vi "configure.vi"(8 "error in (no error)":errorcluster, 11 "WriteSignalsDAQmxPlugin in":refnum<class "SignalWriterDL090202DAQmx.lvclass">) -> (0 "error out":errorcluster, 3 "WriteSignalsDAQmxPlugin out":refnum<class "SignalWriterDL090202DAQmx.lvclass">)   [LabVIEW 2010, in "SignalWriterDL090202DAQmx.lvclass"]
uses:
  SignalWriterDL090202DAQmx.lvclass
  output_type_enum.ctl
  trigger_edge_enum.ctl
  common/classes/GenericComponent/GenericComponent/GenericComponent.lvclass
panel:
  in  "counter":tag
  out "configuration":string
  in  "edge":T1
  in  "digital trigger line":tag
  in  "output value upper bound":dbl caption="to"
  in  "output value  lower bound":dbl caption="from"
  in  "output type":T2
  in  "maximum sampling rate":dbl[unit]
  in  "lag":dbl[unit]
  in  "timing source":tag
  in  "output physical channel":tag
  in  "cancel button":bool
  in  "save button":bool
  # "Configure DL090202DAQmxWriteSignals"
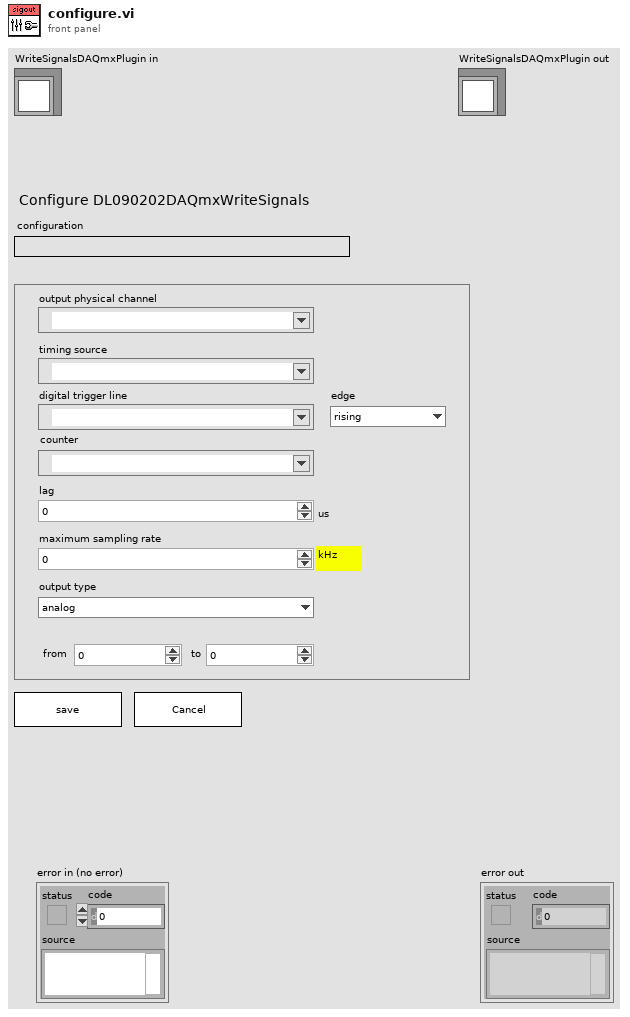
[diagram p1: front panel]
types:
  T1 = typedef "SignalWriterDL090202DAQmx.lvclass/trigger_edge_enum.ctl" = enum16{"rising", "falling"}
  T2 = typedef "SignalWriterDL090202DAQmx.lvclass/output_type_enum.ctl" = enum16{"analog", "digital (U8)", "digital (U16)", "digital (U32)"}
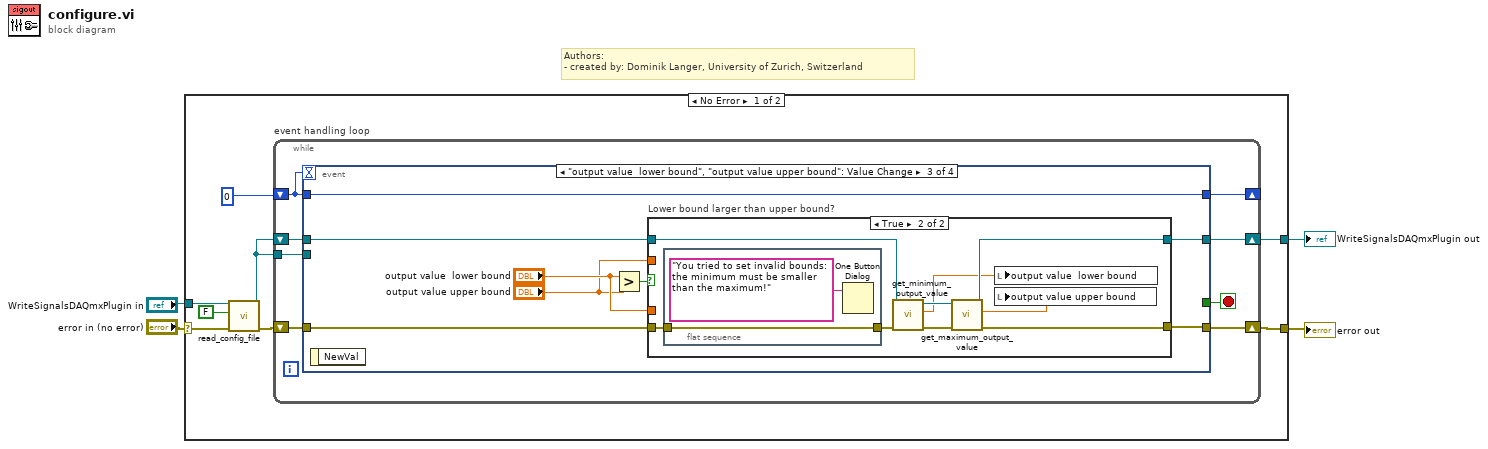
[diagram p0: block diagram]
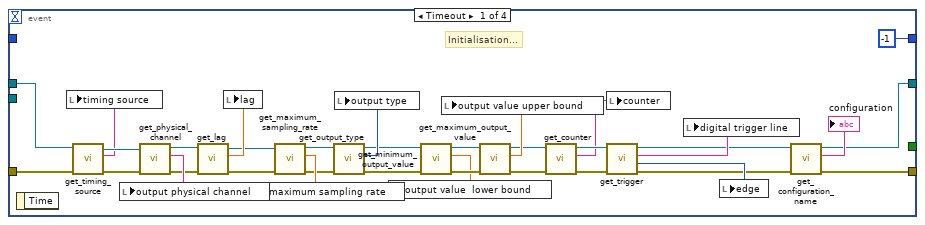
[diagram p2: hidden frame]
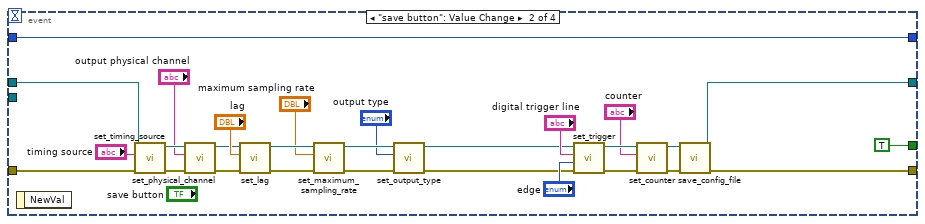
[diagram p3: hidden frame]
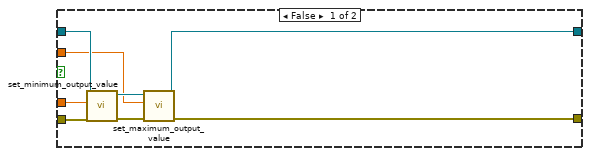
[diagram p4: hidden frame]
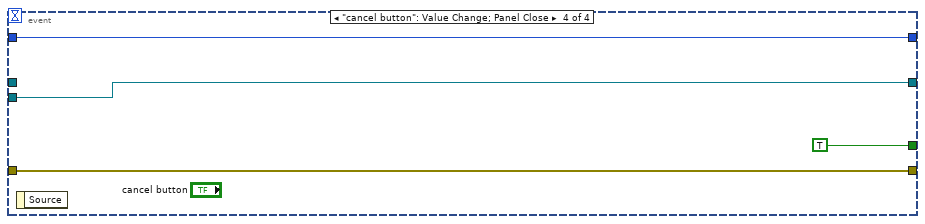
[diagram p5: hidden frame]
diagram:
  # "Authors: \n- created by: Dominik Langer, University of Zurich, Switzerland"
  n1 = case shown="No Error" "error in (no error)" {
    selector: "error in (no error)" -> [w8 w115]
    tunnel: [w12 w115] -> w3
    tunnel: [w10 w114] -> w1
    tunnel: "WriteSignalsDAQmxPlugin in" -> [w9 w114]
    frame No Error {
      n2 = call-dynamic "read_config_file.vi"("error in (no error)"=w8, "force load?"=FALSE, "GenericPlugin in"=w9) -> ("error out"=w7:errorcluster, "GenericPlugin out"=w5:refnum<class "SignalWriterDL090202DAQmx.lvclass">)  [unwired: 7 out]
      n3 = while "event handling loop" {
        shift-right: [w16] -> _
        shift-left: 0 -> [w17]
        shift-right: [w14] -> w10
        shift-left: w5 -> [w15]
        shift-right: [w19] -> w12
        shift-left: w7 -> [w20]
        tunnel: w5 -> [w13]
        stop <- w18 stop-if-true
        n4 = event shown="[2] \"output value  lower bound\", \"output value upper bound\": Value Change" {
          selector: _ -> [_ _ _ _]
          dyn-events: _ -> [_ _ _ _]
          timeout: w17 -> [_ _ _ _]
          tunnel: w20 -> [w34 w79 w89 w112]
          tunnel: [w29 w65 w88 w112] -> w19
          tunnel: [_ TRUE _ TRUE] -> w18
          tunnel: [-1 w82 w90 w111] -> w16
          tunnel: w17 -> [_ w82 w90 w111]
          tunnel: w15 -> [w33 w78 w87 _]
          tunnel: [w26 w64 w86 w110] -> w14
          tunnel: w13 -> [_ _ _ w110]
          event Timeout {
            # "Initialisation..."
            n5 = event-data() -> ()  [unwired: 2 out]
            n6 = call-dynamic "get_timing_source.vi"("error in (no error)"=w34, "DAQmxWriteSignals.lvclass in"=w33) -> ("error out"=w52:errorcluster, "timing source"=w51:tag, "DAQmxWriteSignals.lvclass out"=w53:refnum<class "SignalWriterDL090202DAQmx.lvclass">)  [unwired: 7 out]
            n7 = local write "timing source"(w51) -> ()
            n8 = call-dynamic "get_physical_channel.vi"("error in (no error)"=w52, "DAQmxWriteSignals.lvclass in"=w53) -> ("error out"=w48:errorcluster, "physical channel"=w50:tag, "DAQmxWriteSignals.lvclass out"=w49:refnum<class "SignalWriterDL090202DAQmx.lvclass">)  [unwired: 7 out]
            n9 = local write "output physical channel"(w50) -> ()
            n10 = call-dynamic "get_lag.vi"("error in (no error)"=w48, "GenericWriteSignals.lvclass in"=w49) -> ("error out"=w46:errorcluster, "lag"=w47:dbl[unit], "GenericWriteSignals.lvclass out"=w45:refnum<class "SignalWriterDL090202DAQmx.lvclass">)  [unwired: 7 out]
            n11 = local write "lag"(w47) -> ()
            n12 = call-dynamic "get_maximum_sampling_rate.vi"("error in (no error)"=w46, "DAQmxWriteSignals.lvclass in"=w45) -> ("error out"=w43:errorcluster, "maximum sampling rate"=w44:dbl[unit], "DAQmxWriteSignals.lvclass out"=w42:refnum<class "SignalWriterDL090202DAQmx.lvclass">)  [unwired: 7 out]
            n13 = local write "maximum sampling rate"(w44) -> ()
            n14 = call-dynamic "get_output_type.vi"("error in (no error)"=w43, "DAQmxWriteSignals.lvclass in"=w42) -> ("error out"=w40:errorcluster, "output type"=w41:T2, "DAQmxWriteSignals.lvclass out"=w39:refnum<class "SignalWriterDL090202DAQmx.lvclass">)  [unwired: 7 out]
            n15 = local write "output type"(w41) -> ()
            n16 = call-dynamic "get_minimum_output_value.vi"("error in (no error)"=w40, "GenericWriteSignals.lvclass in"=w39) -> ("error out"=w38:errorcluster, "minimum output value"=w35:dbl, "GenericWriteSignals.lvclass out"=w37:refnum<class "SignalWriterDL090202DAQmx.lvclass">)  [unwired: 7 out]
            n17 = local write "output value  lower bound"(w35) -> ()
            n18 = call-dynamic "get_maximum_output_value.vi"("error in (no error)"=w38, "GenericWriteSignals.lvclass in"=w37) -> ("error out"=w25:errorcluster, "maximum output value"=w36:dbl, "GenericWriteSignals.lvclass out"=w23:refnum<class "SignalWriterDL090202DAQmx.lvclass">)  [unwired: 7 out]
            n19 = local write "output value upper bound"(w36) -> ()
            n20 = call-dynamic "get_counter.vi"("error in (no error)"=w25, "SignalWriterDL090202DAQmx in"=w23) -> ("error out"=w24:errorcluster, "counter"=w21:tag, "SignalWriterDL090202DAQmx out"=w22:refnum<class "SignalWriterDL090202DAQmx.lvclass">)  [unwired: 6 in, 1 out]
            n21 = local write "counter"(w21) -> ()
            n22 = call-dynamic "get_trigger.vi"("error in (no error)"=w24, "DAQmxWriteSignals in"=w22) -> ("error out"=w30:errorcluster, "edge"=w32:T1, "digital trigger line"=w31:tag, "DAQmxWriteSignals out"=w27:refnum<class "SignalWriterDL090202DAQmx.lvclass">)  [unwired: 6 out]
            n23 = local write "digital trigger line"(w31) -> ()
            n24 = local write "edge"(w32) -> ()
            n25 = call "get_configuration_name.vi"("error in (no error)"=w30, "GenericPlugin.lvclass in"=w27) -> ("error out"=w29:errorcluster, "configuration name"=→"configuration":string, "GenericPlugin.lvclass out"=w26:refnum<class "SignalWriterDL090202DAQmx.lvclass">)  [unwired: 7 in]
          }
          event "save button": Value Change {
            n26 = event-data() -> ()  [unwired: 2 out]
            n27 = call-dynamic "set_timing_source.vi"("error in (no error)"=w79, "timing source"="timing source", "DAQmxWriteSignals.lvclass in"=w78) -> ("error out"=w80:errorcluster, "DAQmxWriteSignals.lvclass out"=w77:refnum<class "SignalWriterDL090202DAQmx.lvclass">)  [unwired: 7 out]
            n28 = call-dynamic "set_physical_channel.vi"("error in (no error)"=w80, "physical channel"="output physical channel", "DAQmxWriteSignals.lvclass in"=w77) -> ("error out"=w74:errorcluster, "DAQmxWriteSignals.lvclass out"=w72:refnum<class "SignalWriterDL090202DAQmx.lvclass">)  [unwired: 7 out]
            n29 = call-dynamic "set_lag.vi"("error in (no error)"=w74, "lag"="lag", "DAQmxWriteSignals.lvclass in"=w72) -> ("error out"=w71:errorcluster, "DAQmxWriteSignals.lvclass out"=w70:refnum<class "SignalWriterDL090202DAQmx.lvclass">)  [unwired: 7 out]
            n30 = call-dynamic "set_maximum_sampling_rate.vi"("error in (no error)"=w71, "maximum sampling rate"="maximum sampling rate", "DAQmxWriteSignals.lvclass in"=w70) -> ("error out"=w67:errorcluster, "DAQmxWriteSignals.lvclass out"=w68:refnum<class "SignalWriterDL090202DAQmx.lvclass">)  [unwired: 7 out]
            n31 = call-dynamic "set_output_type.vi"("error in (no error)"=w67, "output type"="output type", "DAQmxWriteSignals.lvclass in"=w68) -> ("error out"=w56:errorcluster, "DAQmxWriteSignals.lvclass out"=w55:refnum<class "SignalWriterDL090202DAQmx.lvclass">)  [unwired: 7 out]
            n32 = call-dynamic "set_trigger.vi"("error in (no error)"=w56, "edge"="edge", "digital trigger line"="digital trigger line", "DAQmxWriteSignals in"=w55) -> ("error out"=w61:errorcluster, "DAQmxWriteSignals out"=w59:refnum<class "SignalWriterDL090202DAQmx.lvclass">)  [unwired: 6 out]
            n33 = call-dynamic "set_counter.vi"("error in (no error)"=w61, "counter"="counter", "SignalWriterDL090202DAQmx in"=w59) -> ("error out"=w60:errorcluster, "SignalWriterDL090202DAQmx out"=w58:refnum<class "SignalWriterDL090202DAQmx.lvclass">)  [unwired: 7 in]
            n34 = call-dynamic "save_config_file.vi"("error in (no error)"=w60, "GenericPlugin in"=w58) -> ("error out"=w65:errorcluster, "GenericPlugin out"=w64:refnum<class "SignalWriterDL090202DAQmx.lvclass">)  [unwired: 2 in, 6 out]
          }
          event "output value  lower bound", "output value upper bound": Value Change {
            n35 = event-data() -> ()  [unwired: 2 out]
            n36 = Greater?(x="output value  lower bound", y="output value upper bound") -> (0:w85:bool)
            n37 = case "Lower bound larger than upper bound?" shown="True" w85 {
              tunnel: w89 -> [w97 w100]
              tunnel: [w95 w105] -> w88
              tunnel: w87 -> [w94 w104]
              tunnel: [w93 w103] -> w86
              tunnel: "output value  lower bound" -> [w92 _]
              tunnel: "output value upper bound" -> [w91 _]
              frame False {
                n38 = call-dynamic "set_minimum_output_value.vi"("error in (no error)"=w97, "minimum output value"=w92, "DAQmxWriteSignals.lvclass in"=w94) -> ("error out"=w96:errorcluster, "DAQmxWriteSignals.lvclass out"=w98:refnum<class "SignalWriterDL090202DAQmx.lvclass">)  [unwired: 7 out]
                n39 = call-dynamic "set_maximum_output_value.vi"("error in (no error)"=w96, "maximum output value"=w91, "DAQmxWriteSignals.lvclass in"=w98) -> ("error out"=w95:errorcluster, "DAQmxWriteSignals.lvclass out"=w93:refnum<class "SignalWriterDL090202DAQmx.lvclass">)  [unwired: 7 out]
              }
              frame True {
                n40 = flat-sequence {
                  tunnel: w100 -> [w109]
                  tunnel: [w109] -> w99
                  frame #0 {
                    n41 = One Button Dialog(message="You tried to set invalid bounds: the minimum must be smaller than the maximum!") -> ()  [unwired: 1 in, 1 out]
                  }
                }
                n42 = call-dynamic "get_minimum_output_value.vi"("error in (no error)"=w99, "GenericWriteSignals.lvclass in"=w104) -> ("error out"=w106:errorcluster, "minimum output value"=w102:dbl, "GenericWriteSignals.lvclass out"=w107:refnum<class "SignalWriterDL090202DAQmx.lvclass">)  [unwired: 7 out]
                n43 = call-dynamic "get_maximum_output_value.vi"("error in (no error)"=w106, "GenericWriteSignals.lvclass in"=w107) -> ("error out"=w105:errorcluster, "maximum output value"=w101:dbl, "GenericWriteSignals.lvclass out"=w103:refnum<class "SignalWriterDL090202DAQmx.lvclass">)  [unwired: 7 out]
                n44 = local write "output value  lower bound"(w102) -> ()
                n45 = local write "output value upper bound"(w101) -> ()
              }
            }
          }
          event "cancel button": Value Change; Panel Close {
            n46 = event-data() -> ()  [unwired: 2 out]
          }
        }
      }
    }
    frame Error {
    }
  }
  "error out" <- w3
  "WriteSignalsDAQmxPlugin out" <- w1
